vi "op_biti_v2.vi"() -> ()   [LabVIEW 2010]
panel:
  in  "Numeric 10":u8=255
  out "Array":bool[](array[boolean])=[FALSE, FALSE, FALSE, FALSE, FALSE, TRUE, FALSE, TRUE]
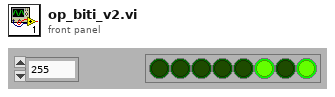
[diagram p1: front panel]
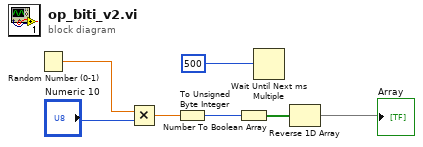
[diagram p0: block diagram]
diagram:
  n1 = Random Number (0-1)() -> (number: 0 to 1=w6:dbl)
  n2 = Multiply(x=w6, y="Numeric 10") -> (x*y=w2:dbl)
  n3 = To Unsigned Byte Integer(number=w2) -> (unsigned 8bit integer=w1:u8)
  n4 = Number To Boolean Array(number=w1) -> (Boolean array=w5:bool[])
  n5 = Wait Until Next ms Multiple(millisecond multiple=500) -> ()  [unwired: 1 out]
  n6 = Reverse 1D Array(array=w5) -> (reversed array=→"Array":bool[])
